vi "Set Disabled.vi"(8 "error in (no error)":errorcluster, 10 "Disabled":bool, 11 "GuiLinkButton in":refnum<class "GuiLinkButton.lvclass">) -> (0 "error out":errorcluster, 3 "GuiLinkButton out":refnum<class "GuiLinkButton.lvclass">)   [LabVIEW 2020, in "VolatusGUIElements.lvlib" / "GuiLinkButton.lvclass"]
uses:
  GuiLinkButton.lvclass
  GuiLinkButton.lvclass/GuiLinkButton.ctl
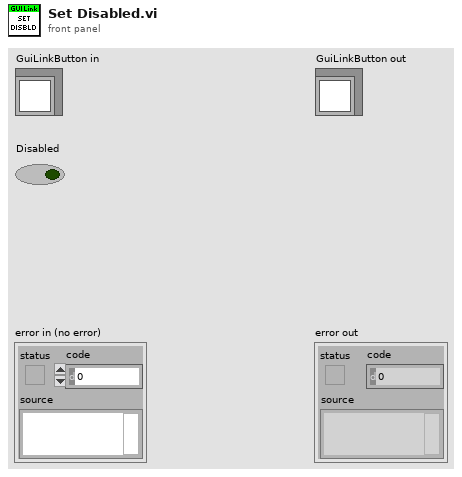
[diagram p1: front panel]
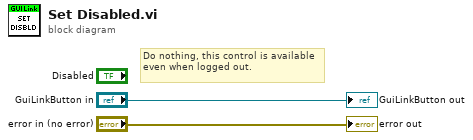
[diagram p0: block diagram]
diagram:
  # "Do nothing, this control is available even when logged out."
  "error out" <- "error in (no error)"
  "GuiLinkButton out" <- "GuiLinkButton in"
